vi "StatusCalculation.vi"(1 "ProductionBoard":T1={"StartHour"=[{"Hour"=5, "Minute"=0}, {"Hour"=6, "Minute"=0}, {"Hour"=7, "Minute"=0}, {"Hour"=7, "Minute"=30}, {"Hour"=0, "Minute"=0}, {"Hour"=0, "Minute"=0}, {"Hour"=0, "Minute"=0}, {"Hour"=0, "Minute"=0}, {"Hour"=0, "Minute"=0}], "Goal"=[], "EndHour"=[{"Hour"=5, "Minute"=59}, {"Hour"=6, "Minute"=59}, {"Hour"=7, "Minute"=10}, {"Hour"=7, "Minute"=59}, {"Hour"=0, "Minute"=0}, {"Hour"=0, "Minute"=0}, {"Hour"=0, "Minute"=0}, {"Hour"=0, "Minute"=0}, {"Hour"=0, "Minute"=0}], "AM/PM"=[{"AM/PM"=0}, {"AM/PM"=0}, {"AM/PM"=0}, {"AM/PM"=0}, {"AM/PM"=0}, {"AM/PM"=0}, {"AM/PM"=0}, {"AM/PM"=0}, {"AM/PM"=0}], "Actual"=[], "%"=[], "Status"=[], "Comments"=[]} caption="ProductionBoardIN" {"AM/PM"."AM/PM" items=["AM", "PM"]; "EndHour"."Minute" items=["00", "1", "2", "3", "4", "5", "6", "7", "8", "9", "10", "11", "12", "13", "14", "15", "16", "17", "18", "19", "20", "21", "22", "23", "24", "25", "26", "27", "28", "29", "30", "31", "32", "33", "34", "35", "36", "37", "38", "39", "40", "41", "42", "43", "44", "45", "46", "47", "48", "49", "50", "51", "52", "53", "54", "55", "56", "57", "58", "59"]; "EndHour"."Hour" items=["00", "1", "2", "3", "4", "5", "6", "7", "8", "9", "10", "11", "12", "13", "14", "15", "16", "17", "18", "19", "20", "21", "22", "23"]; "StartHour"."Minute" items=["00", "1", "2", "3", "4", "5", "6", "7", "8", "9", "10", "11", "12", "13", "14", "15", "16", "17", "18", "19", "20", "21", "22", "23", "24", "25", "26", "27", "28", "29", "30", "31", "32", "33", "34", "35", "36", "37", "38", "39", "40", "41", "42", "43", "44", "45", "46", "47", "48", "49", "50", "51", "52", "53", "54", "55", "56", "57", "58", "59"]; "StartHour"."Hour" items=["00", "1", "2", "3", "4", "5", "6", "7", "8", "9", "10", "11", "12", "13", "14", "15", "16", "17", "18", "19", "20", "21", "22", "23"]}) -> (0 "ProductionBoard 2":T1={"StartHour"=[{"Hour"=5, "Minute"=0}, {"Hour"=6, "Minute"=0}, {"Hour"=7, "Minute"=0}, {"Hour"=7, "Minute"=30}, {"Hour"=0, "Minute"=0}, {"Hour"=0, "Minute"=0}, {"Hour"=0, "Minute"=0}, {"Hour"=0, "Minute"=0}, {"Hour"=0, "Minute"=0}], "Goal"=[], "EndHour"=[{"Hour"=5, "Minute"=59}, {"Hour"=6, "Minute"=59}, {"Hour"=7, "Minute"=10}, {"Hour"=7, "Minute"=59}, {"Hour"=0, "Minute"=0}, {"Hour"=0, "Minute"=0}, {"Hour"=0, "Minute"=0}, {"Hour"=0, "Minute"=0}, {"Hour"=0, "Minute"=0}], "AM/PM"=[{"AM/PM"=0}, {"AM/PM"=0}, {"AM/PM"=0}, {"AM/PM"=0}, {"AM/PM"=0}, {"AM/PM"=0}, {"AM/PM"=0}, {"AM/PM"=0}, {"AM/PM"=0}], "Actual"=[], "%"=[], "Status"=[], "Comments"=[]} caption="ProductionBoardOUT" {"AM/PM"."AM/PM" items=["AM", "PM"]; "EndHour"."Minute" items=["00", "1", "2", "3", "4", "5", "6", "7", "8", "9", "10", "11", "12", "13", "14", "15", "16", "17", "18", "19", "20", "21", "22", "23", "24", "25", "26", "27", "28", "29", "30", "31", "32", "33", "34", "35", "36", "37", "38", "39", "40", "41", "42", "43", "44", "45", "46", "47", "48", "49", "50", "51", "52", "53", "54", "55", "56", "57", "58", "59"]; "EndHour"."Hour" items=["00", "1", "2", "3", "4", "5", "6", "7", "8", "9", "10", "11", "12", "13", "14", "15", "16", "17", "18", "19", "20", "21", "22", "23"]; "StartHour"."Minute" items=["00", "1", "2", "3", "4", "5", "6", "7", "8", "9", "10", "11", "12", "13", "14", "15", "16", "17", "18", "19", "20", "21", "22", "23", "24", "25", "26", "27", "28", "29", "30", "31", "32", "33", "34", "35", "36", "37", "38", "39", "40", "41", "42", "43", "44", "45", "46", "47", "48", "49", "50", "51", "52", "53", "54", "55", "56", "57", "58", "59"]; "StartHour"."Hour" items=["00", "1", "2", "3", "4", "5", "6", "7", "8", "9", "10", "11", "12", "13", "14", "15", "16", "17", "18", "19", "20", "21", "22", "23"]})   [LabVIEW 2017]
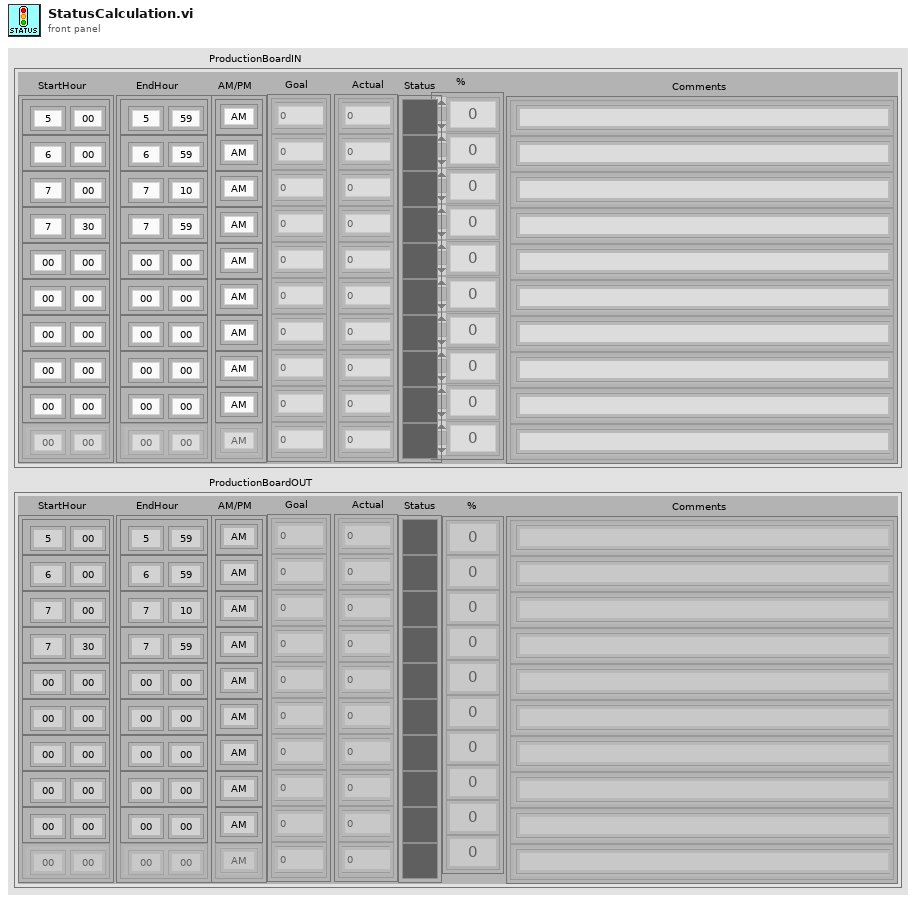
[diagram p1: front panel]
types:
  T1 = cluster{"StartHour":cluster{"Hour":u16, "Minute":u16}[], "Goal":cluster{"Goal":dbl}[], "EndHour":cluster{"Hour":u16, "Minute":u16}[], "AM/PM":cluster{"AM/PM":u16}[], "Actual":cluster{"Actual":dbl}[], "%":i32[], "Status":u32[], "Comments":cluster{"Comments":string}[]}
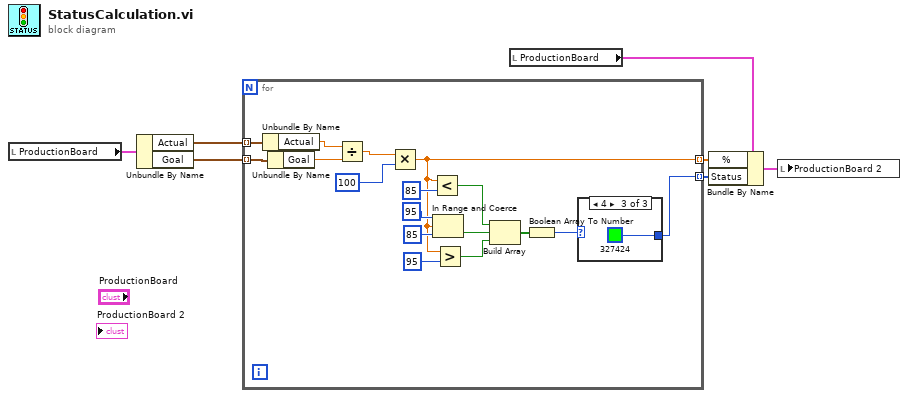
[diagram p0: block diagram]
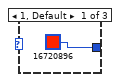
[diagram p2: hidden frame]
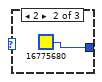
[diagram p3: hidden frame]
diagram:
  n1 = local read "ProductionBoard"() -> (w7:T1)
  n2 = Unbundle By Name(w7) -> ("Actual"=w6:cluster{"Actual":dbl}[], "Goal"=w5:cluster{"Goal":dbl}[])
  n3 = for {
    tunnel: w6 -> [w24] mode=indexing
    tunnel: w5 -> [w23] mode=indexing
    tunnel: [w14] -> w3 mode=indexing
    tunnel: [w8] -> w1 mode=indexing
    n4 = Unbundle By Name(w24) -> ("Actual"=w21:dbl)
    n5 = Unbundle By Name(w23) -> ("Goal"=w22:dbl)
    n6 = Divide(x=w21, y=w22) -> (x/y=w20:dbl)
    n7 = Multiply(x=w20, y=100) -> (x*y=w14:dbl)
    n8 = Less?(x=w14, y=85) -> (x < y?=w13:bool)
    n9 = In Range and Coerce(upper limit=95, x=w14, lower limit=85) -> (In Range?=w12:bool)  [unwired: 1 out]
    n10 = Greater?(x=w14, y=95) -> (0:w11:bool)
    n11 = Build Array(w13, w12, w11) -> (w10:bool[])
    n12 = Boolean Array To Number(Boolean array=w10) -> (number=w9:u32)
    n13 = case shown="4" w9 {
      tunnel: [u32 16720896 u32 16775680 u32 327424] -> w8
      frame 1, Default {
      }
      frame 2 {
      }
      frame 4 {
      }
    }
  }
  n14 = local read "ProductionBoard"() -> (w4:T1)
  n15 = Bundle By Name(cluster=w4, "%"=w3, "Status"=w1) -> (w2:T1)
  n16 = local write "ProductionBoard 2"(w2) -> ()
